vi "Add Documentation to Deconstructor VI.vi"   [LabVIEW 2015]
doc: "<b> </b> <b> </b>\n©2016 Q Software Innovations, LLC (QSI)\nwritten by Quentin Alldredge\nproduced in LabVIEW 2015"
uses:
  Project Manipulation Scripts/Project Manipulation Scripts.lvlib
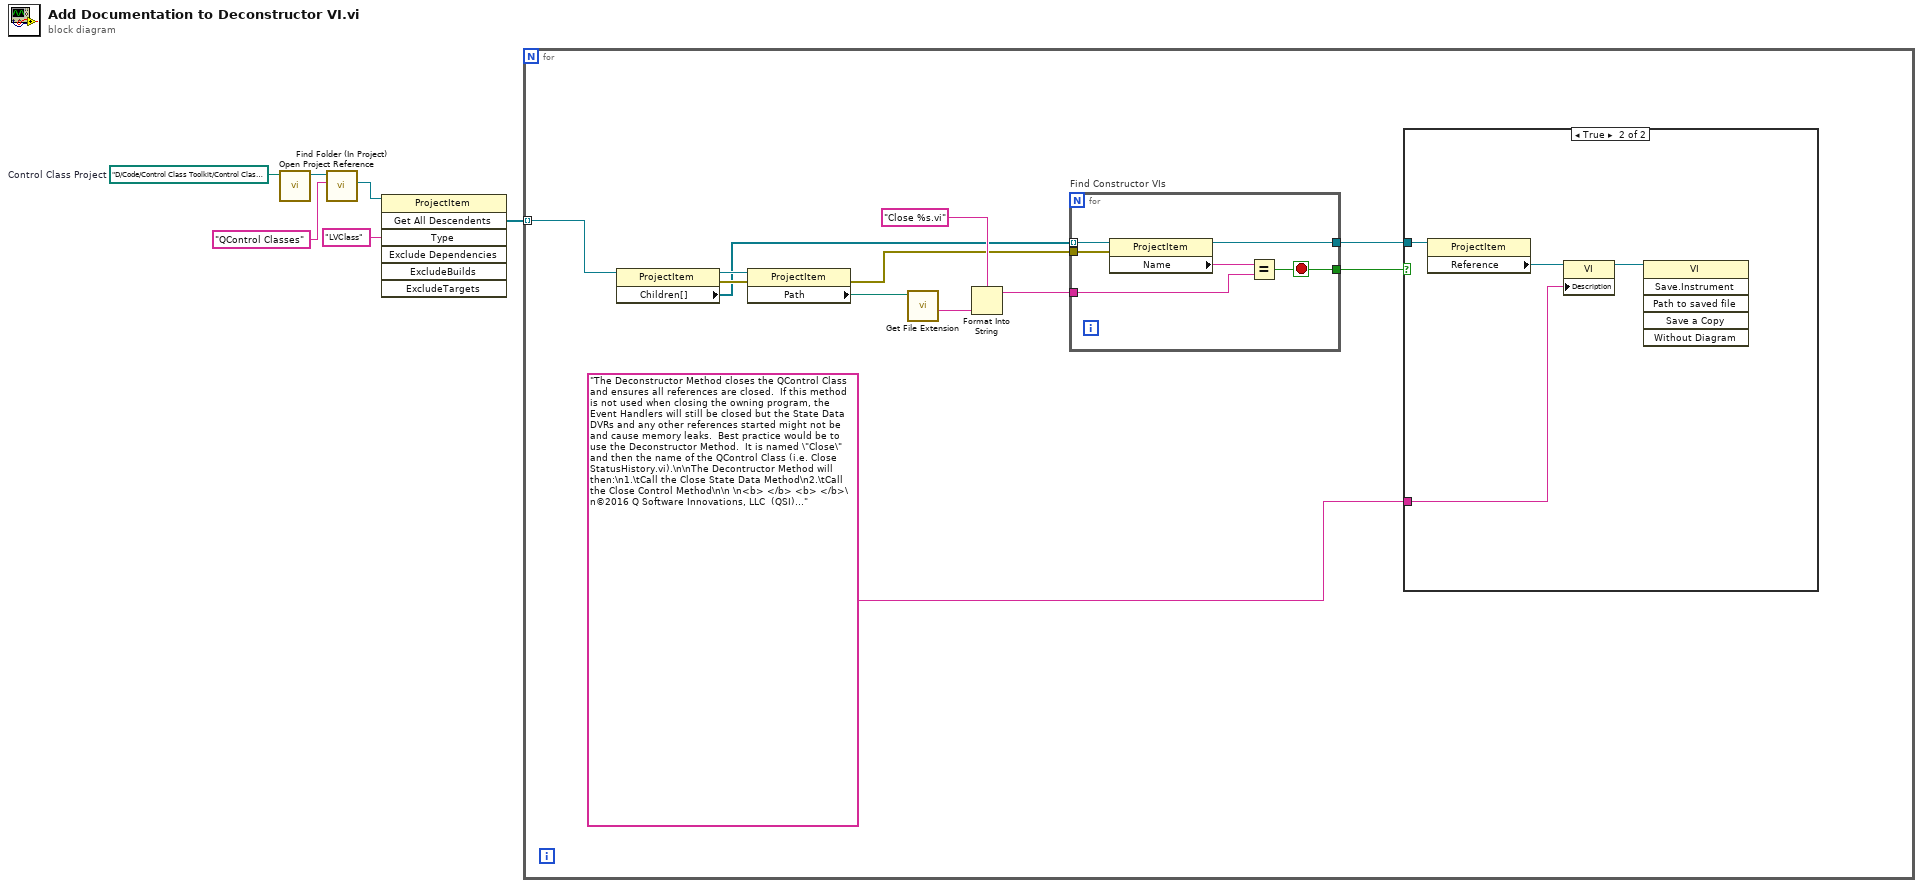
[diagram p0: block diagram]
diagram:
  w6 = path "D:/Code/Control Class Toolkit/Control Class Toolkit.lvproj"  # Control Class Project
  n1 = call "Open Project Reference.vi"("Project Path"=w6) -> ("Project out"=w5:refnum<vi>)  [unwired: 10 in]
  n2 = call "Find Folder (In Project).vi"("Folder Name"="QControl Classes", "Project in"=w5) -> ("Folder Refnum"=w3:refnum<vi>)  [unwired: 7 in, 2 out]
  n3 = invoke class="ProjectItem" method="Get All Descendents"(reference=w3, "Type"="LVClass") -> ("All Descendents"=w1:refnum<vi>[])  [unwired: 5 in, 6 out]
  n4 = for {
    tunnel: w1 -> [w16] mode=indexing
    n5 = property class="ProjectItem"(reference=w16) -> (reference out=w14:refnum<vi>, error out=w9:errorcluster, "Children[]"=w7:refnum<vi>[])  [unwired: 1 in]
    n6 = property class="ProjectItem"(reference=w14, error in=w9) -> (error out=w8:errorcluster, "Path"=w13:path)  [unwired: 1 out]
    n7 = call <vilib>:"Get File Extension.vi"("file"=w13) -> ("filename without extension"=w11:string)  [unwired: 6 in, 4 out]
    n8 = Format Into String(format string="Close %s.vi", w11) -> (resulting string=w10:string)  [unwired: 2 in, 1 out]
    n9 = for "Find Constructor VIs" {
      tunnel: w8 -> [w20]
      tunnel: [w24] -> w17
      tunnel: [w21] -> w18
      tunnel: w10 -> [w22]
      tunnel: w7 -> [w19] mode=indexing
      stop <- w21 stop-if-true
      n10 = property class="ProjectItem"(reference=w19, error in=w20) -> (reference out=w24:refnum<vi>, "Name"=w23:string)  [unwired: 1 out]
      n11 = Equal?(x=w23, y=w22) -> (x = y?=w21:bool)
    }
    n12 = case shown="True" w18 {
      tunnel: w17 -> [_ w28]
      tunnel: "The Deconstructor Method closes the QControl Class and ensures all references are closed.  If this method is not used when closing the owning program, the Event Handlers will still be closed but the State Data DVRs and any other references started might not be and cause memory leaks.  Best practice would be to use the Deconstructor Method.  It is named \"Close\" and then the name of the QControl Class (i.e. Close StatusHistory.vi).\n\nThe Decontructor Method will then:\n1.\tCall the Close State Data Method\n2.\tCall the Close Control Method\n\n \n<b> </b> <b> </b>\n©2016 Q Software Innovations, LLC  (QSI)\nwritten by Quentin Alldredge\nproduced in LabVIEW 2015 " ("VI Description") -> [_ w26]
      frame False {
      }
      frame True {
        n13 = property class="ProjectItem"(reference=w28) -> ("Reference"=w27:refnum<vi>)  [unwired: 1 in, 2 out]
        n14 = property class="VI"(reference=w27, "Description"=w26) -> (reference out=w25:refnum<vi>)  [unwired: 1 in, 1 out]
        n15 = invoke class="VI" method="Save.Instrument"(reference=w25) -> ()  [unwired: 5 in, 6 out]
      }
    }
  }
